vi "ep_Speed Calculation.vi"(0 "harmonic frequency":dbl, 1 "fundamental frequency [Hz]":dbl format="%#_13g", 5 "pole pairs":i32, 7 "harmonic for speed calculation":i32, 9 "range of speed":T2, 11 "error in (no error)":errorcluster) -> (4 "speed data":cluster{"speed [RPM]":dbl, "slip":dbl}={"speed [RPM]"=nan, "slip"=nan}, 8 "harmonic for speed calculation":T1, 15 "error out":errorcluster)   [LabVIEW 2014, in "NI_EP_Motor Monitoring.lvlib"]
uses:
  <vilib>/addons/Electrical Power/Motor Monitoring/NI_EP_Motor Monitoring.lvlib
  <vilib>/addons/Electrical Power/Motor Monitoring/subVIs/ep_Harmonic for Speed Calculation.ctl
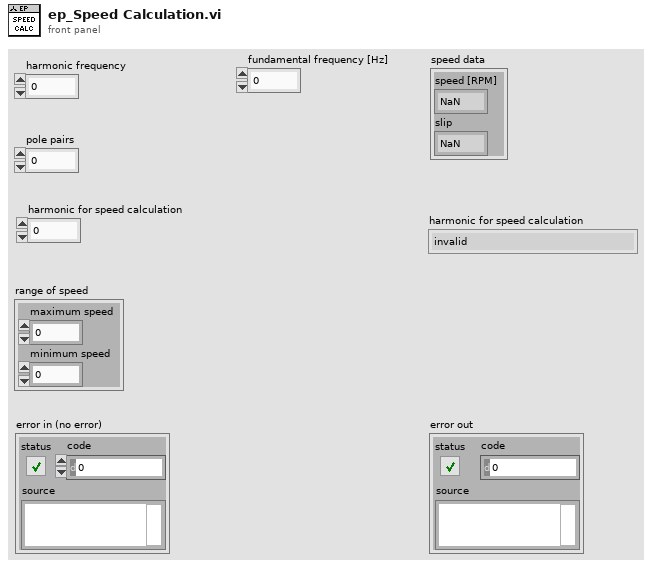
[diagram p1: front panel]
types:
  T1 = typedef "NI_EP_Motor Monitoring.lvlib/ep_Harmonic for Speed Calculation.ctl" = enum16{"invalid", "fr", "2fs-2fr", "2fs-fr", "2fr"}
  T2 = cluster{"maximum speed":dbl, "minimum speed":dbl}
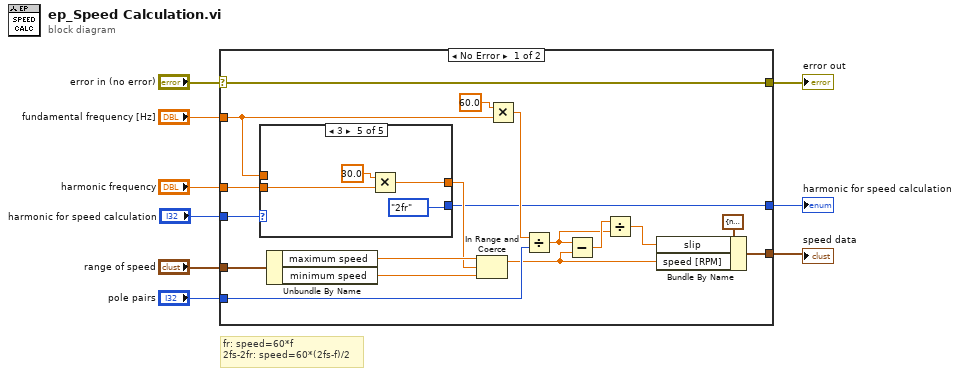
[diagram p0: block diagram]
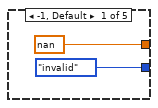
[diagram p2: hidden frame]
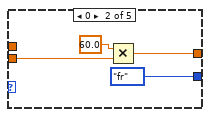
[diagram p3: hidden frame]
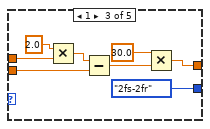
[diagram p4: hidden frame]
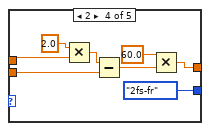
[diagram p5: hidden frame]
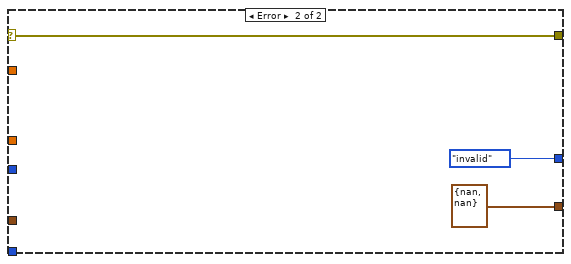
[diagram p6: hidden frame]
diagram:
  # "fr: speed=60*f\n2fs-2fr: speed=60*(2fs-f)/2"
  n1 = case shown="No Error" "error in (no error)" {
    selector: "error in (no error)" -> [w27 w56]
    tunnel: "fundamental frequency [Hz]" -> [w14 _]
    tunnel: [w27 w56] -> w7
    tunnel: "pole pairs" -> [w24 _]
    tunnel: [w19 cluster{"speed [RPM]":dbl, "slip":dbl} {"speed [RPM]"=nan, "slip"=nan} ("speed data")] -> w5
    tunnel: "range of speed" -> [w18 _]
    tunnel: "harmonic frequency" -> [w15 _]
    tunnel: [w11 ep_Harmonic_for_Speed_Calculation."invalid" ("harmonic for speed calculation")] -> w2
    tunnel: "harmonic for speed calculation" -> [w10 _]
    frame No Error {
      n2 = case shown="3" w10 {
        tunnel: w15 -> [_ w32 w35 w44 w52]
        tunnel: [nan ("y") w31 w39 w43 w51] -> w13
        tunnel: w14 -> [_ _ w41 w45 _]
        tunnel: [ep_Harmonic_for_Speed_Calculation."invalid" ep_Harmonic_for_Speed_Calculation."fr" ("harmonic for speed calculation") ep_Harmonic_for_Speed_Calculation."2fs-2fr" ("harmonic for speed calculation") ep_Harmonic_for_Speed_Calculation."2fs-fr" ("harmonic for speed calculation") ep_Harmonic_for_Speed_Calculation."2fr" ("harmonic for speed calculation")] -> w11
        frame -1, Default {
        }
        frame 0 {
          n3 = Multiply(x=60.0 ("y"), y=w32) -> (x*y=w31:dbl)
        }
        frame 1 {
          n4 = Multiply(x=2.0, y=w41) -> (x*y=w36:dbl)
          n5 = Subtract(x=w36, y=w35) -> (x-y=w37:dbl)
          n6 = Multiply(x=30.0 ("y"), y=w37) -> (x*y=w39:dbl)
        }
        frame 2 {
          n7 = Multiply(x=2.0, y=w45) -> (x*y=w48:dbl)
          n8 = Subtract(x=w48, y=w44) -> (x-y=w46:dbl)
          n9 = Multiply(x=60.0 ("y"), y=w46) -> (x*y=w43:dbl)
        }
        frame 3 {
          n10 = Multiply(x=30.0 ("y"), y=w52) -> (x*y=w51:dbl)
        }
      }
      n11 = Unbundle By Name(w18) -> ("maximum speed"=w17:dbl, "minimum speed"=w16:dbl)
      n12 = In Range and Coerce(upper limit=w17, x=w13, lower limit=w16) -> (coerced(x)=w12:dbl)  [unwired: 1 out]
      n13 = Multiply(x=60.0 ("y"), y=w14) -> (x*y=w25:dbl)
      n14 = Divide(x=w25, y=w24) -> (x/y=w22:dbl)
      n15 = Subtract(x=w22, y=w12) -> (x-y=w23:dbl)
      n16 = Divide(x=w23, y=w22) -> (x/y=w20:dbl)
      n17 = Bundle By Name(cluster=cluster{"speed [RPM]":dbl, "slip":dbl} {"speed [RPM]"=nan, "slip"=nan} ("speed data"), "slip"=w20, "speed [RPM]"=w12) -> (w19:cluster{"speed [RPM]":dbl, "slip":dbl})
    }
    frame Error {
    }
  }
  "error out" <- w7
  "speed data" <- w5
  "harmonic for speed calculation" <- w2
